vi "SC TCP Read Data.vi"(6 "timeout ms (25000)":i32=25000, 8 "error in":errorcluster, 11 "TCP  Connection in":refnum<k5>) -> (0 "error out":errorcluster, 2 "data":string, 3 "TCP  Connection out":refnum<k5>)   [LabVIEW 2018]
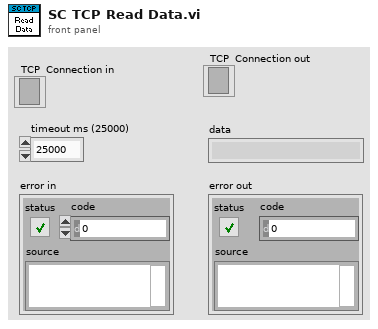
[diagram p1: front panel]
types:
  T1 = enum16{"Standard", "Buffered", "CRLF", "Immediate"}
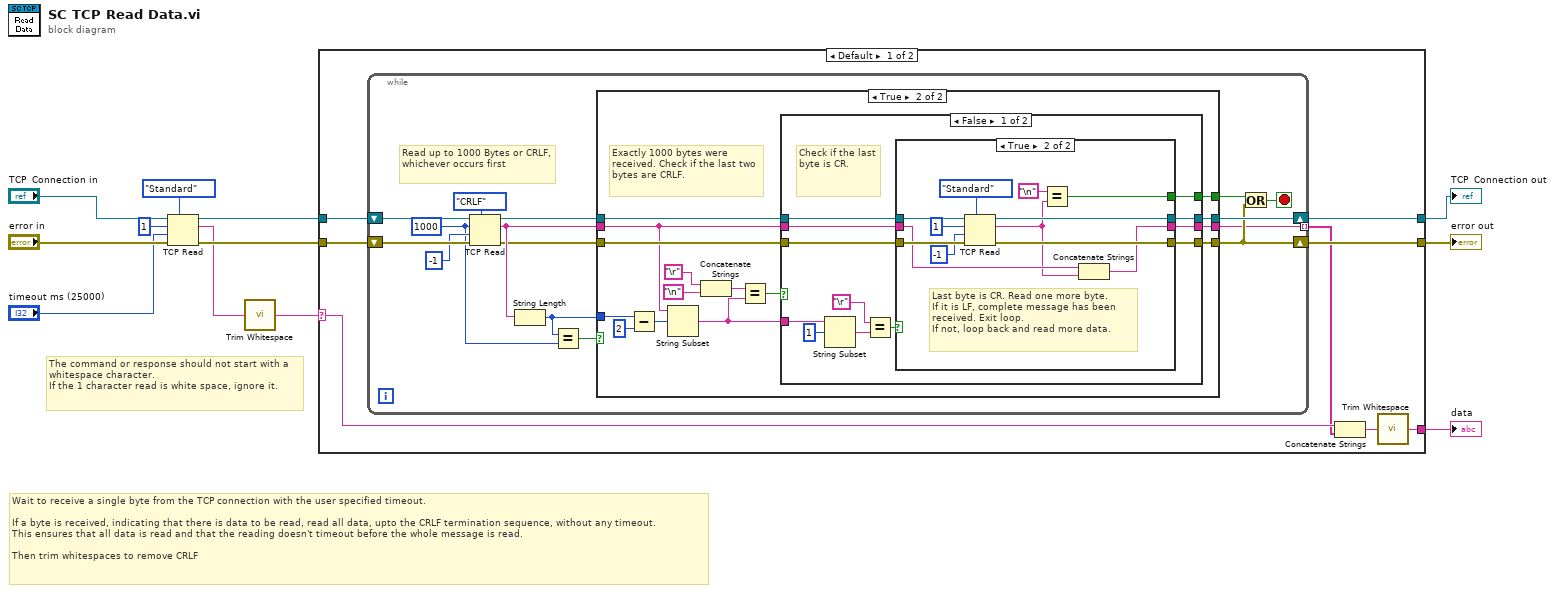
[diagram p0: block diagram]
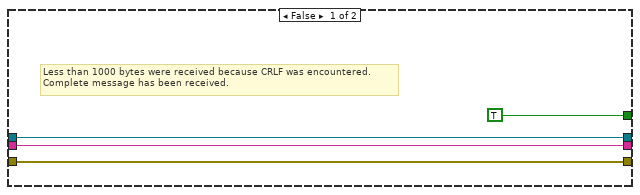
[diagram p2: hidden frame]
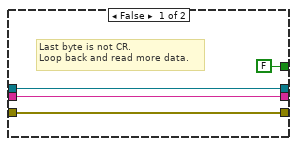
[diagram p3: hidden frame]
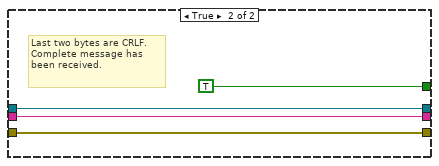
[diagram p4: hidden frame]
diagram:
  # "The command or response should not start with a whitespace character.\nIf the 1 character read is white space, ignore it."
  # "Wait to receive a single byte from the TCP connection with the user specified timeout.\n\nIf a byte is received, indicating that there is data to be read, read all data, upto the CRLF termination sequence, without any timeout. \nThis ensures that all data is read and that the reading doesn't timeout before the whole message is read.\n\nThen trim whitespaces to remove CRLF"
  n1 = TCP Read(connection ID="TCP  Connection in", bytes to read=1, error in (no error)="error in", 7:T1."Standard" ("mode (standard)"), 9:"timeout ms (25000)") -> (connection ID out=w6:refnum<k5>, data out=w3:string, error out=w5:errorcluster)
  n2 = call <vilib>:"Trim Whitespace.vi"("string"=w3) -> ("trimmed string"=w2:string)  [unwired: 1 in]
  n3 = case shown="Default" w2 {
    selector: w2 -> [w16 _]
    tunnel: [w20 w87] -> w12
    tunnel: [w19 w88] -> w8
    tunnel: w6 -> [w18 w88]
    tunnel: w5 -> [w17 w87]
    tunnel: [w14 _] -> w11
    frame Default {
      n4 = while {
        tunnel: [w22] -> w13 mode=indexing
        shift-right: [w24] -> w19
        shift-left: w18 -> [w34]
        shift-right: [w23] -> w20
        shift-left: w17 -> [w33]
        stop <- w31 stop-if-true
        w30 = 1000 ("bytes to read")
        # "Read up to 1000 Bytes or CRLF, whichever occurs first"
        n5 = TCP Read(connection ID=w34, bytes to read=w30, error in (no error)=w33, 7:T1."CRLF" ("mode (standard)"), 9:-1 ("timeout ms (25000)")) -> (connection ID out=w25:refnum<k5>, data out=w28:string, error out=w26:errorcluster)
        n6 = String Length(string=w28) -> (length=w27:i32)
        n7 = Equal?(x=w27, y=w30) -> (x = y?=w29:bool)
        n8 = case shown="True" w29 {
          tunnel: w28 -> [w38 w42]
          tunnel: w27 -> [_ w52]
          tunnel: w26 -> [w37 w46]
          tunnel: w25 -> [w39 w45]
          tunnel: [w39 w44] -> w24
          tunnel: [w37 w43] -> w23
          tunnel: [w38 w41] -> w22
          tunnel: [TRUE w40] -> w21
          frame False {
            # "Less than 1000 bytes were received because CRLF was encountered.\nComplete message has been received."
          }
          frame True {
            # "Exactly 1000 bytes were received. Check if the last two bytes are CRLF."
            n9 = Subtract(x=w52, y=2) -> (x-y=w53:i32)
            n10 = String Subset(string=w42, offset (0)=w53) -> (substring=w48:string)  [unwired: 1 in]
            n11 = Concatenate Strings("\r", "\n") -> (w50:string)
            n12 = Equal?(x=w50, y=w48) -> (x = y?=w49:bool)
            n13 = case shown="False" w49 {
              tunnel: w48 -> [w65 _]
              tunnel: w46 -> [w63 w85]
              tunnel: w45 -> [w62 w86]
              tunnel: [w61 w86] -> w44
              tunnel: [w60 w85] -> w43
              tunnel: w42 -> [w56 w84]
              tunnel: [w55 w84] -> w41
              tunnel: [w57 TRUE] -> w40
              frame False {
                # "Check if the last byte is CR."
                n14 = String Subset(string=w65, offset (0)=1) -> (substring=w66:string)  [unwired: 1 in]
                n15 = Equal?(x="\r", y=w66) -> (x = y?=w59:bool)
                n16 = case shown="True" w59 {
                  tunnel: w63 -> [w69 w80]
                  tunnel: w62 -> [w70 w79]
                  tunnel: [w70 w78] -> w61
                  tunnel: [w69 w77] -> w60
                  tunnel: [FALSE w74] -> w57
                  tunnel: w56 -> [w68 w73]
                  tunnel: [w68 w71] -> w55
                  frame False {
                    # "Last byte is not CR.\nLoop back and read more data."
                  }
                  frame True {
                    # "Last byte is CR. Read one more byte.\nIf it is LF, complete message has been received. Exit loop. \nIf not, loop back and read more data."
                    n17 = TCP Read(connection ID=w79, bytes to read=1, error in (no error)=w80, 7:T1."Standard" ("mode (standard)"), 9:-1 ("timeout ms (25000)")) -> (connection ID out=w78:refnum<k5>, data out=w72:string, error out=w77:errorcluster)
                    n18 = Equal?(x="\n", y=w72) -> (x = y?=w74:bool)
                    n19 = Concatenate Strings(w73, w72) -> (w71:string)
                  }
                }
              }
              frame True {
                # "Last two bytes are CRLF.\nComplete message has been received."
              }
            }
          }
        }
        n20 = Or(x=w21, y=w23) -> (x .or. y?=w31:bool)
      }
      n21 = Concatenate Strings(w16, w13) -> (w15:string)
      n22 = call <vilib>:"Trim Whitespace.vi"("string"=w15) -> ("trimmed string"=w14:string)  [unwired: 1 in]
    }
    frame "" {
    }
  }
  "error out" <- w12
  "data" <- w11
  "TCP  Connection out" <- w8
